vi "NF WF1973_74 PHAS Swap.vi"(8 "error in (no error)":errorcluster caption="Error IN", 10 "Ch(Ch1)":bool, 11 "VISAsession":refnum<visa-resource-name>) -> (0 "error out":errorcluster caption="Error OUT", 3 "CopyVISAsession":refnum<visa-resource-name>)   [LabVIEW 2010]
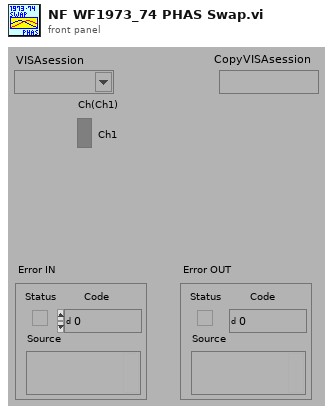
[diagram p1: front panel]
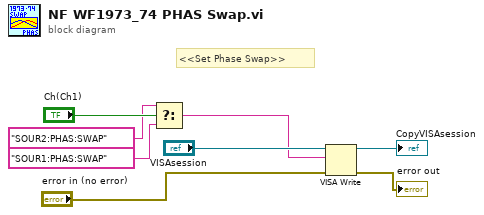
[diagram p0: block diagram]
diagram:
  # "<<Set Phase Swap>>"
  n1 = Select(t="SOUR2:PHAS:SWAP" ("文字列"), s="Ch(Ch1)", f="SOUR1:PHAS:SWAP" ("文字列")) -> (s? t:f=w1:string)
  n2 = VISA Write(VISA resource name="VISAsession", write buffer=w1, error in (no error)="error in (no error)") -> (VISA resource name out=→"CopyVISAsession":refnum<visa-resource-name>, error out=→"error out":errorcluster)  [unwired: 1 out]
